vi "通讯协议解析.vi"(11 "字符串":string) -> (0 "指令":u8[](array[numeric]), 1 "通道地址":u8[](array[numeric]), 2 "帧头":u8[](array[numeric]), 3 "包长度":u8[](array[numeric]))   [LabVIEW 2016]
panel:
  out "子数组 3":u8[](array[numeric])
  out "子数组 2":u8[](array[numeric])
  out "子数组":u8[](array[numeric])
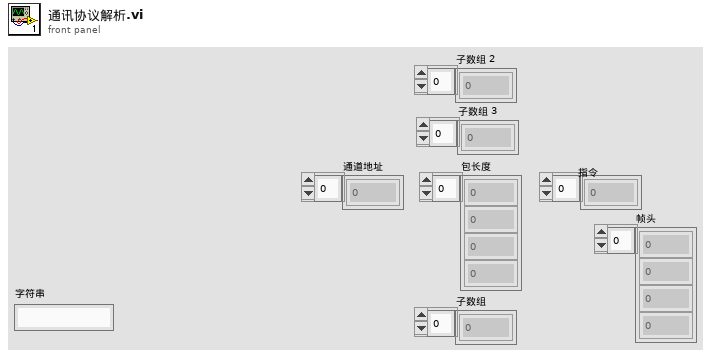
[diagram p1: front panel]
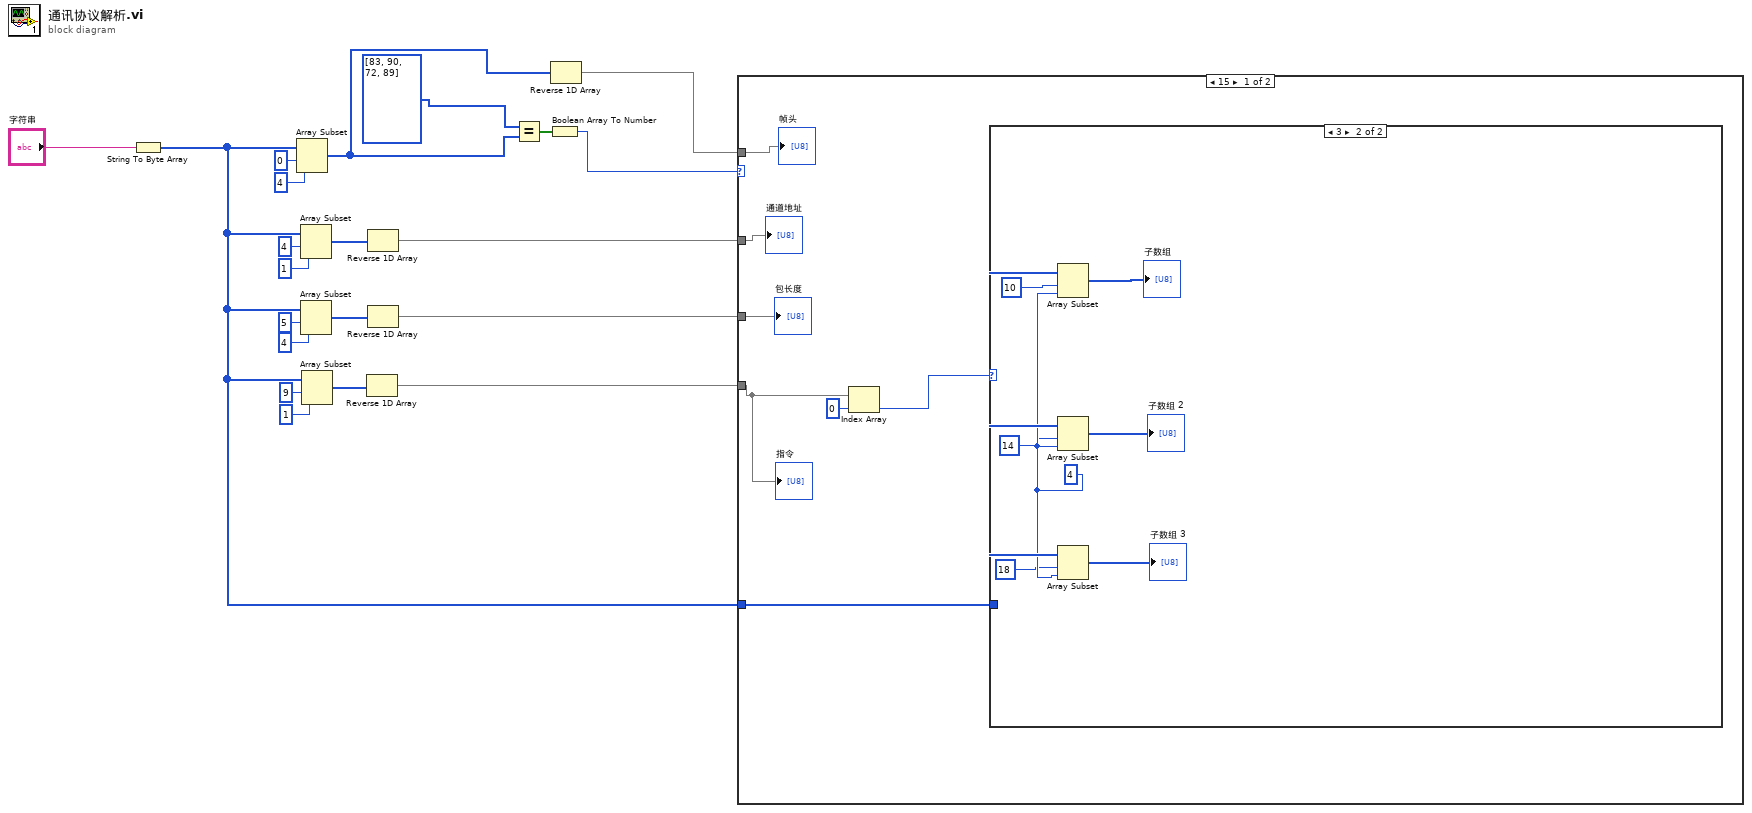
[diagram p0: block diagram]
diagram:
  n1 = String To Byte Array(string="字符串") -> (unsigned byte array=w1:u8[])
  n2 = Array Subset(array=w1, index=0 ("索引"), length=4 ("长度")) -> (w3:u8[])
  n3 = Array Subset(array=w1, index=4 ("索引"), length=1 ("长度")) -> (w12:u8[])
  n4 = Array Subset(array=w1, index=5 ("索引"), length=4 ("长度")) -> (w11:u8[])
  n5 = Array Subset(array=w1, index=9 ("索引"), length=1 ("长度")) -> (w10:u8[])
  n6 = Reverse 1D Array(array=w10) -> (reversed array=w4:u8[])
  n7 = Reverse 1D Array(array=w12) -> (reversed array=w6:u8[])
  n8 = Reverse 1D Array(array=w11) -> (reversed array=w5:u8[])
  n9 = Equal?(x=u8[] [83, 90, 72, 89], y=w3) -> (x = y?=w8:bool[])
  n10 = Boolean Array To Number(Boolean array=w8) -> (number=w7:u32)
  n11 = Reverse 1D Array(array=w3) -> (reversed array=w2:u8[])
  n12 = case shown="15" w7 {
    tunnel: w2 -> [w22 _]
    tunnel: w6 -> [w28 _]
    tunnel: w5 -> [w27 _]
    tunnel: w4 -> [w26 _]
    tunnel: w1 -> [w23 _]
    frame 15 {
      n13 = Index Array(array=w26, index=0 ("索引")) -> (element=w24:u8)
      n14 = case shown="3" w24 {
        tunnel: w23 -> [_ w36]
        frame 0, Default {
        }
        frame 3 {
          w35 = 4 ("长度")
          n15 = Array Subset(array=w36, index=10 ("索引"), length=w35) -> (→"子数组":u8[])
          n16 = Array Subset(array=w36, index=14 ("索引"), length=w35) -> (→"子数组 2":u8[])
          n17 = Array Subset(array=w36, index=18 ("索引"), length=w35) -> (→"子数组 3":u8[])
        }
      }
      "帧头" <- w22
      "通道地址" <- w28
      "包长度" <- w27
      "指令" <- w26
    }
    frame 0, Default {
    }
  }
